vi "Step Forward.vi"(3 "error in":errorcluster, 4 "Data in":T1, 5 "Step control reference in":refnum<vi>) -> (0 "error out":errorcluster, 1 "Data out":T1, 2 "Step control reference out":refnum<vi>)   [LabVIEW 2015]
uses:
  Data.ctl
  Diagnostics.ctl
  Systems.ctl
  Step Vis/Steps.lvlib
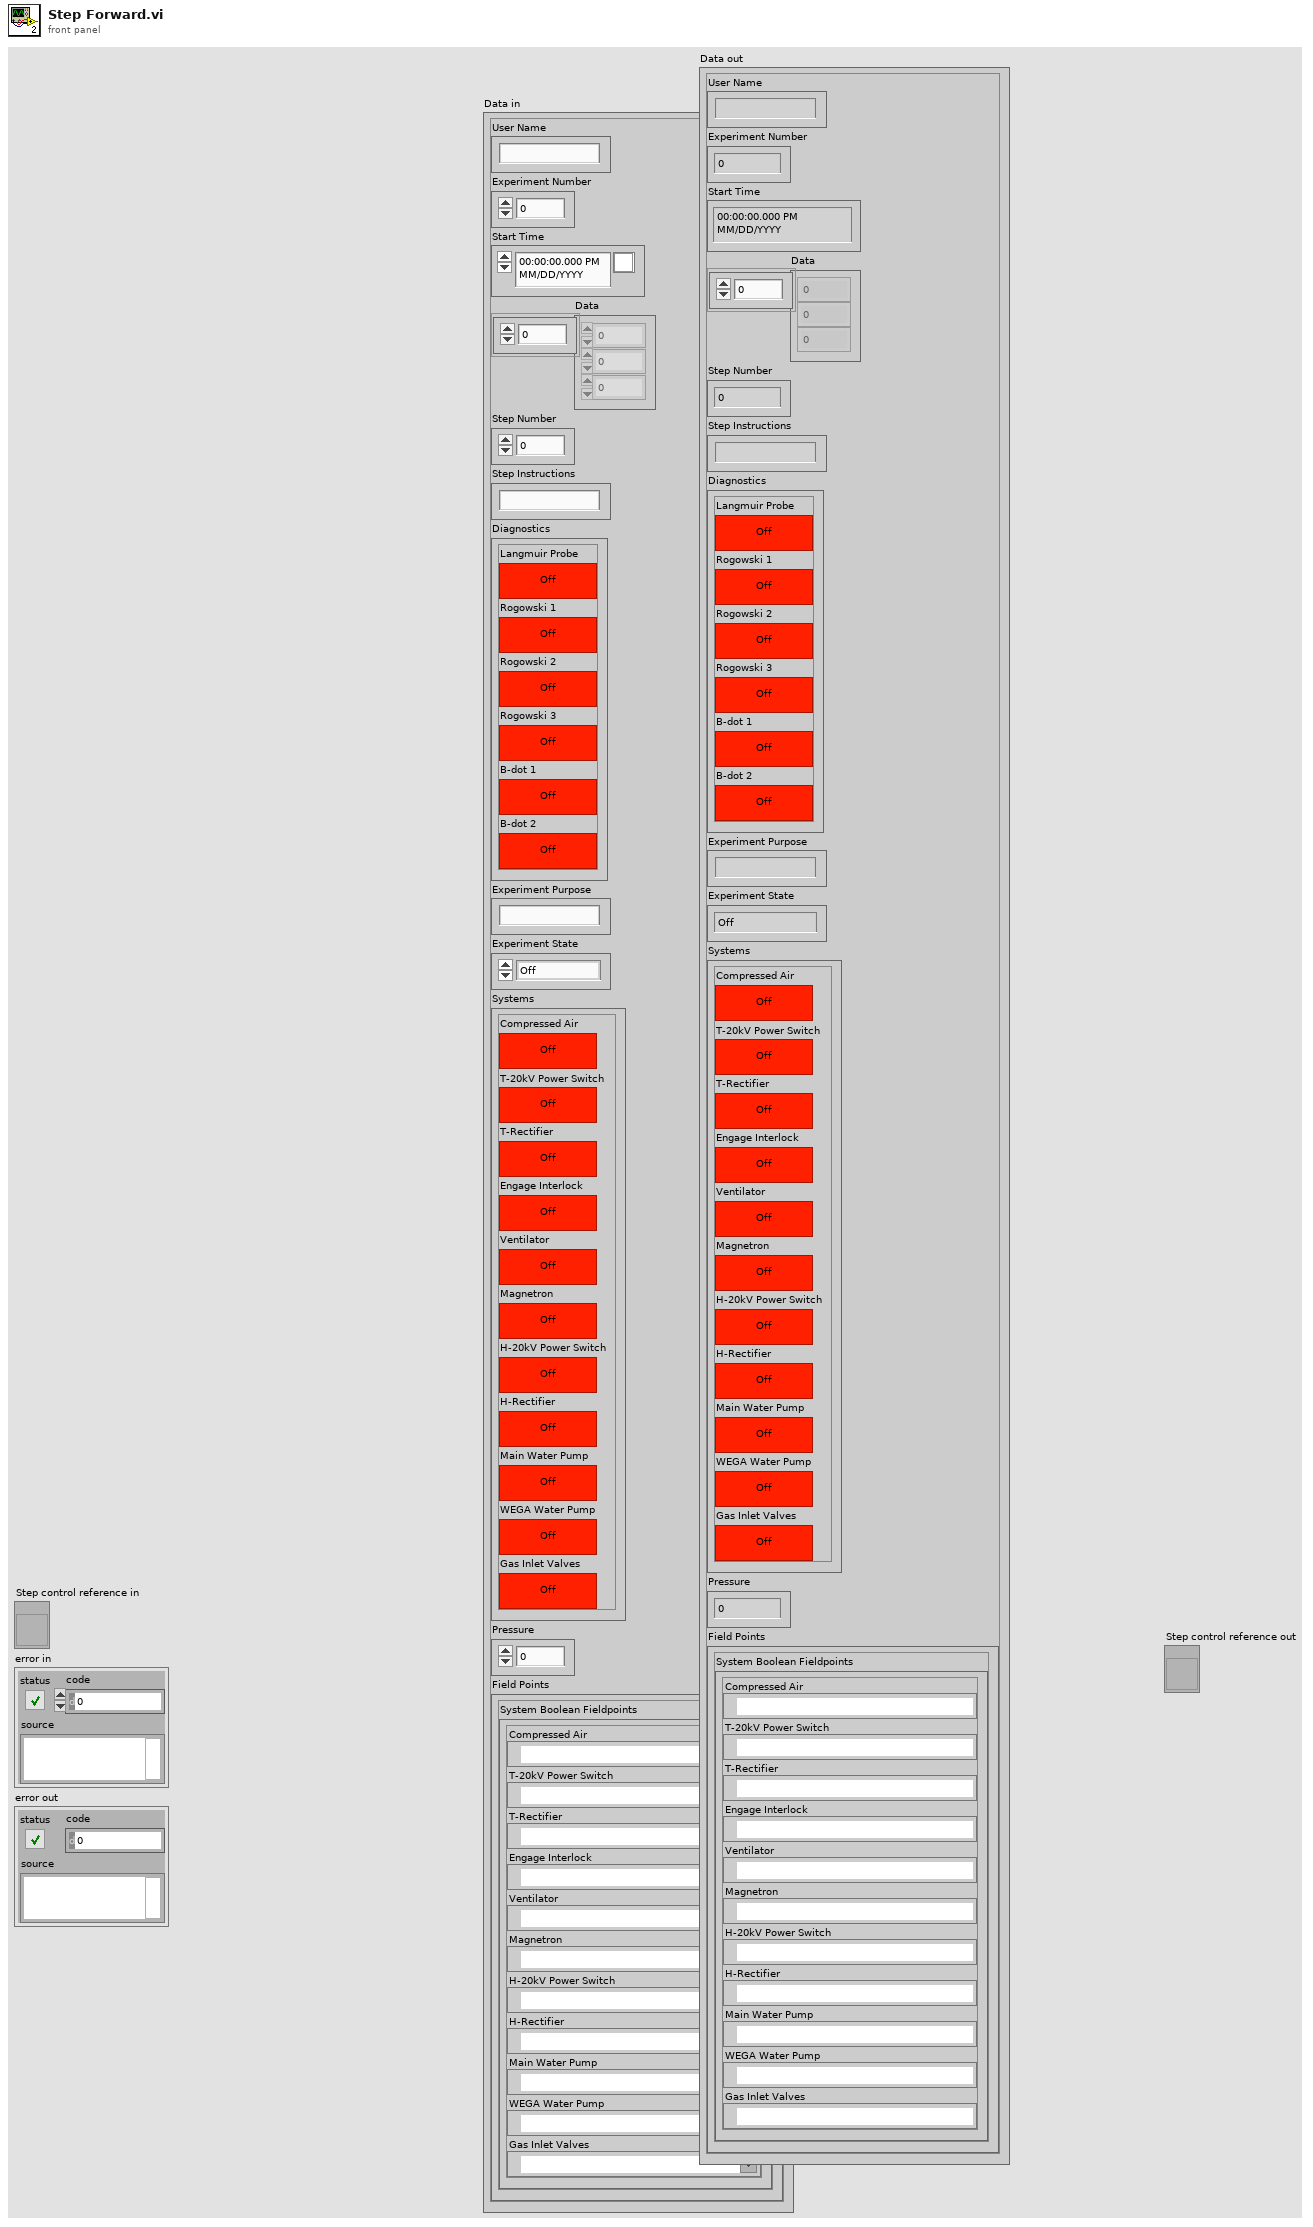
[diagram p1: front panel]
types:
  T1 = typedef "Data.ctl" = cluster{"User Name":string, "Experiment Number":i32, "Start Time":timestamp, "Data":dbl[], "Step Number":i32, "Step Instructions":string, "Diagnostics":T2, "Experiment Purpose":string, "Experiment State":enum16{"Off", "Setting Up", "Ready", "In Progress", "Shutting Down"}, "Systems":T3, "Pressure":dbl, "Field Points":cluster{"System Boolean Fieldpoints":cluster{"Compressed Air":refnum<k21>, "T-20kV Power Switch":refnum<k21>, "T-Rectifier":refnum<k21>, "Engage Interlock":refnum<k21>, "Ventilator":refnum<k21>, "Magnetron":refnum<k21>, "H-20kV Power Switch":refnum<k21>, "H-Rectifier":refnum<k21>, "Main Water Pump":refnum<k21>, "WEGA Water Pump":refnum<k21>, "Gas Inlet Valves":refnum<k21>}}}
  T2 = typedef "Diagnostics.ctl" = cluster{"Langmuir Probe":bool, "Rogowski 1":bool, "Rogowski 2":bool, "Rogowski 3":bool, "B-dot 1":bool, "B-dot 2":bool}
  T3 = typedef "Systems.ctl" = cluster{"Compressed Air":bool, "T-20kV Power Switch":bool, "T-Rectifier":bool, "Engage Interlock":bool, "Ventilator":bool, "Magnetron":bool, "H-20kV Power Switch":bool, "H-Rectifier":bool, "Main Water Pump":bool, "WEGA Water Pump":bool, "Gas Inlet Valves":bool}
  T4 = enum16{"Off", "Setting Up", "Ready", "In Progress", "Shutting Down"}
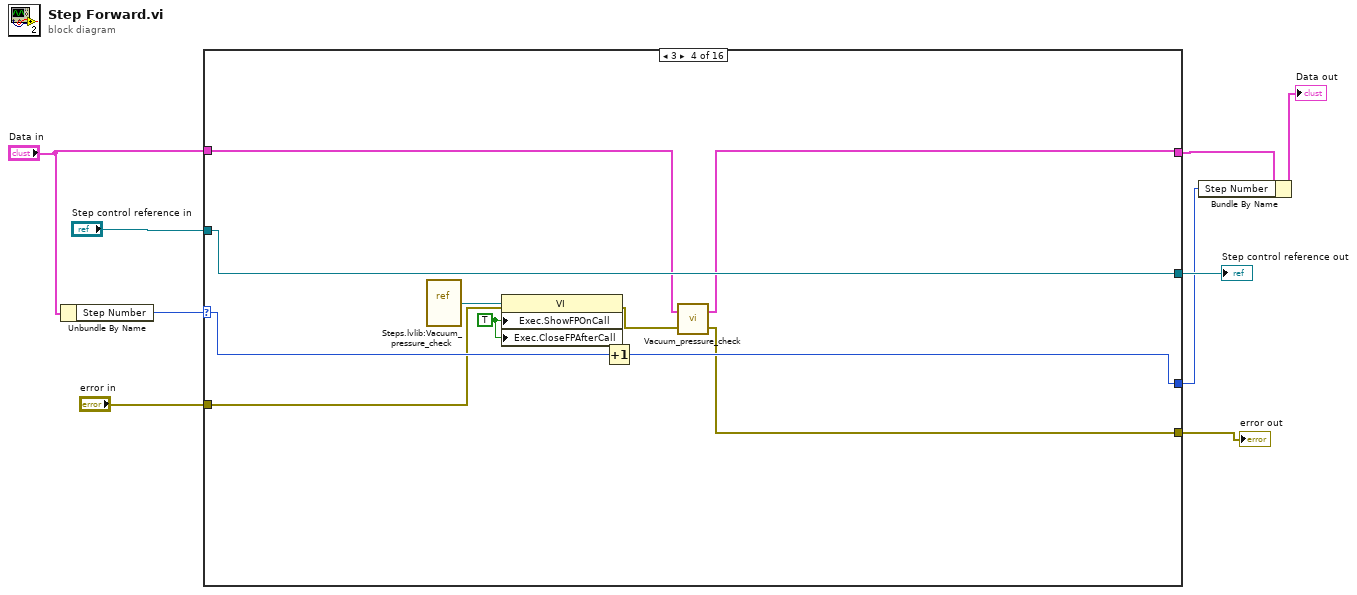
[diagram p0: block diagram]
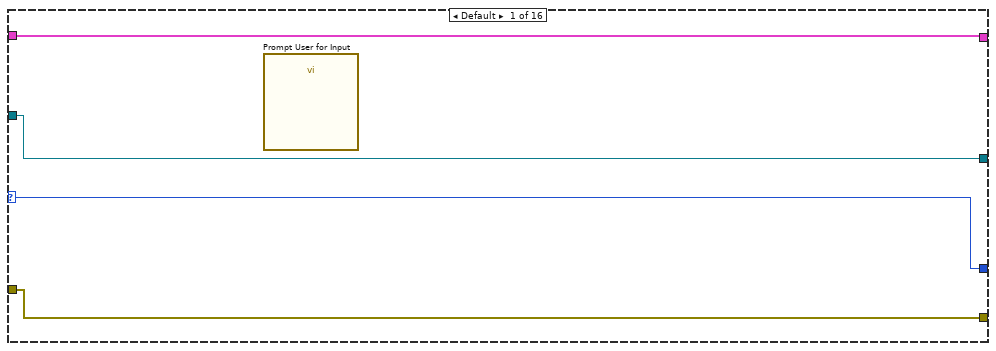
[diagram p2: hidden frame]
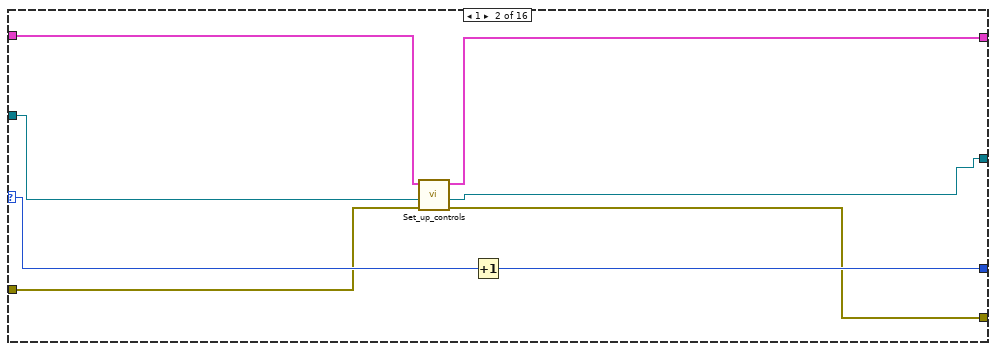
[diagram p3: hidden frame]
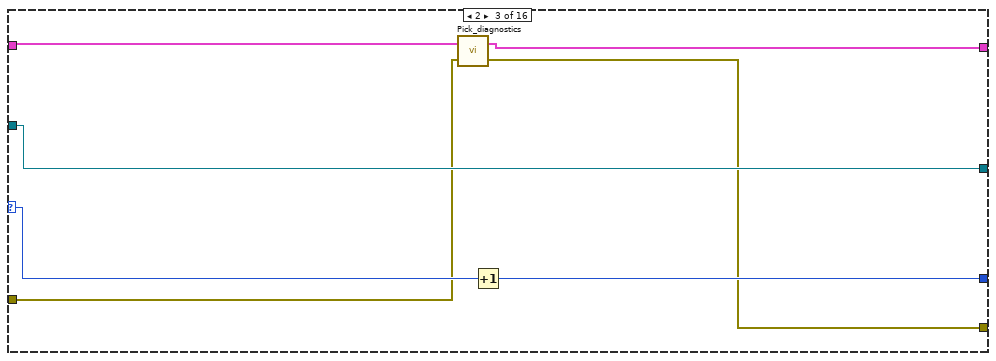
[diagram p4: hidden frame]
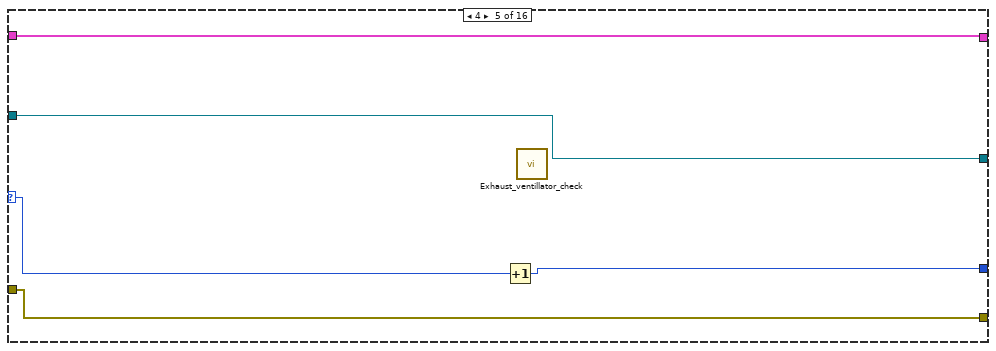
[diagram p5: hidden frame]
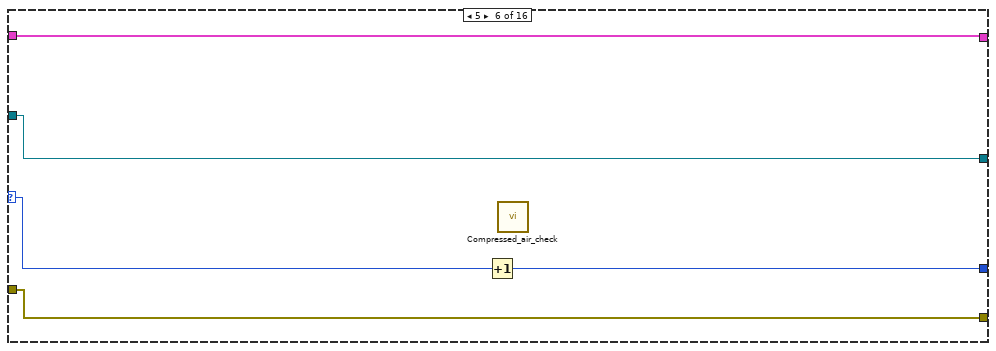
[diagram p6: hidden frame]
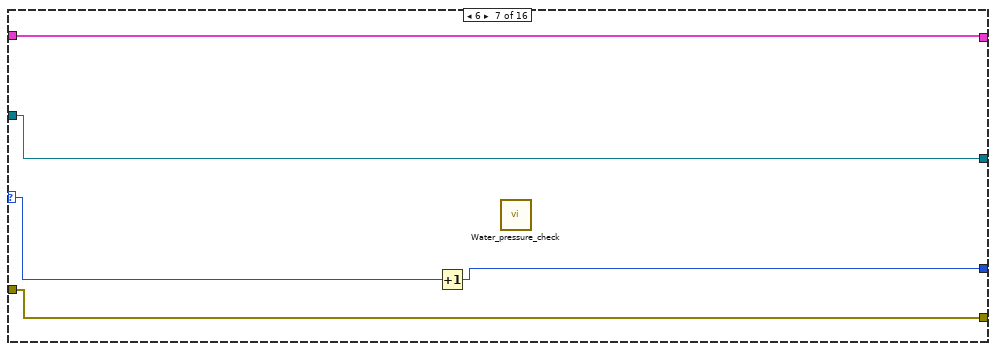
[diagram p7: hidden frame]
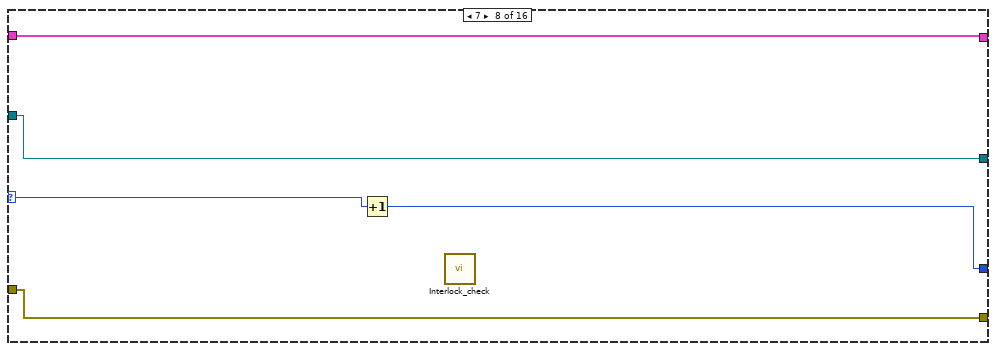
[diagram p8: hidden frame]
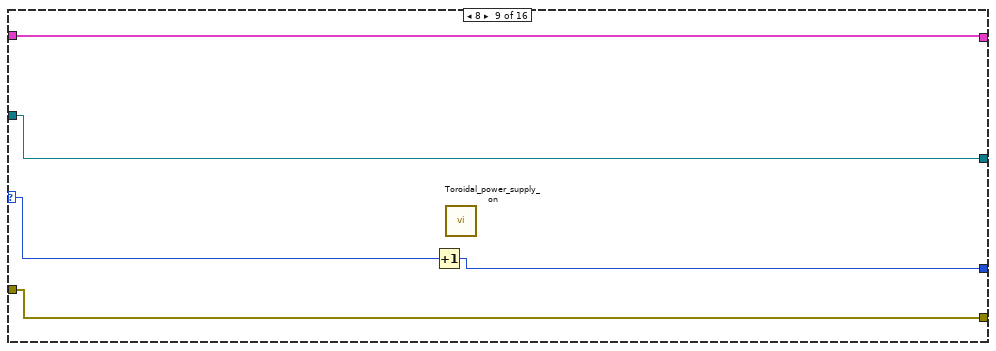
[diagram p9: hidden frame]
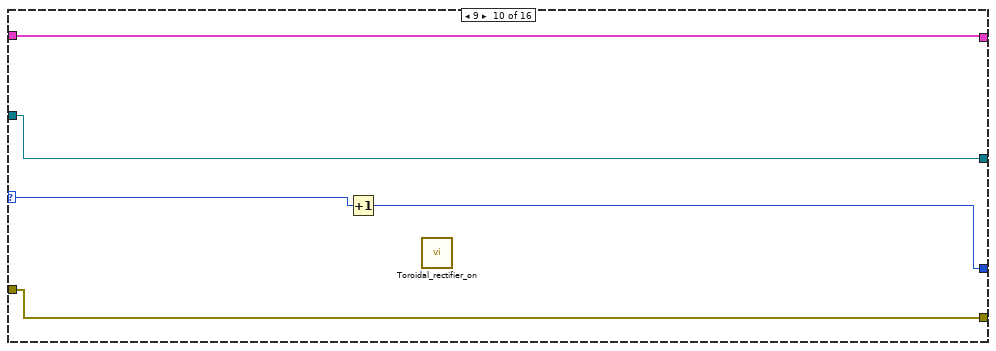
[diagram p10: hidden frame]
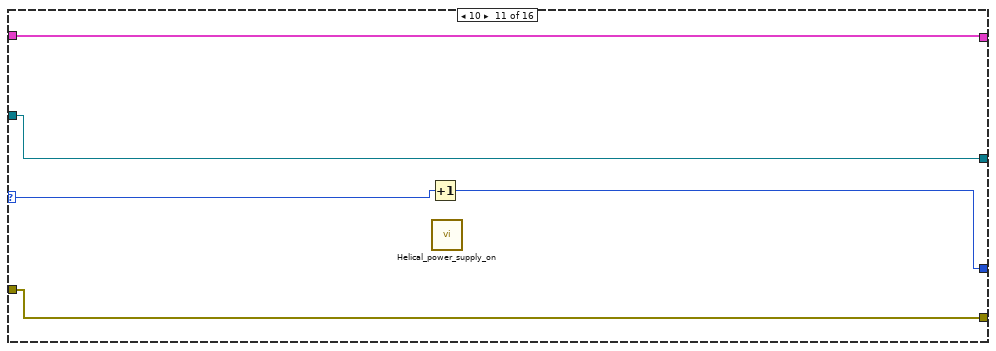
[diagram p11: hidden frame]
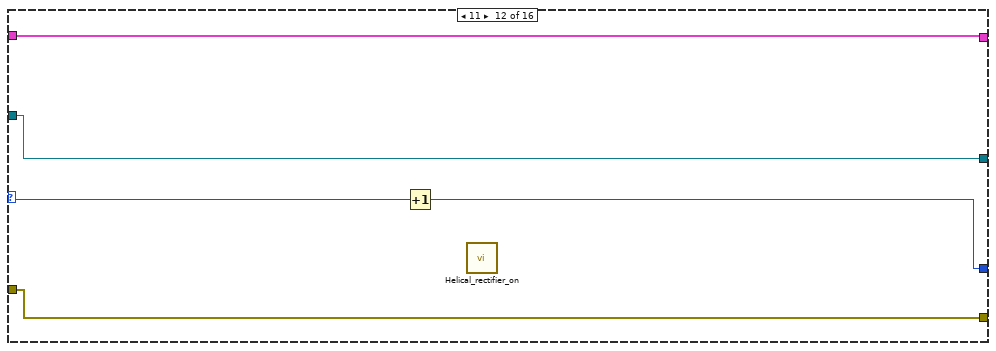
[diagram p12: hidden frame]
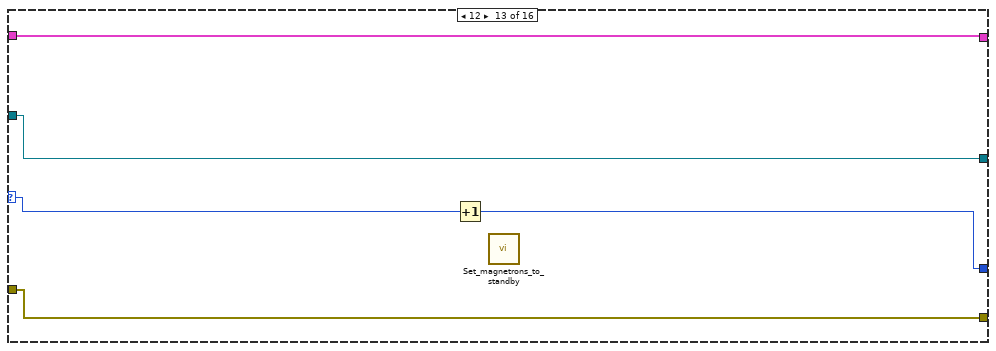
[diagram p13: hidden frame]
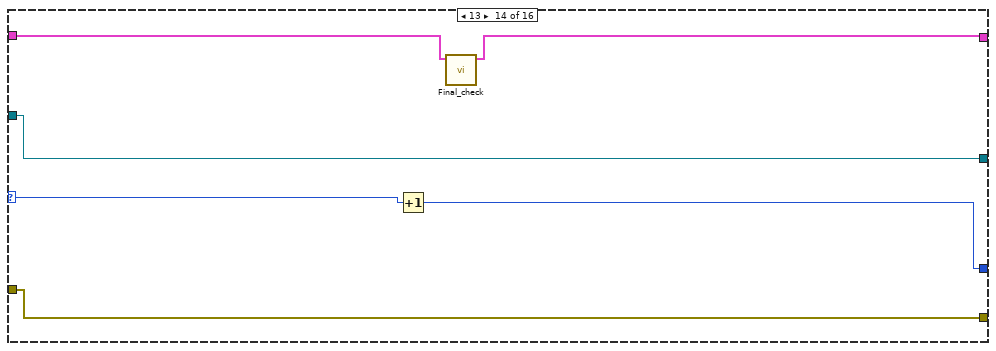
[diagram p14: hidden frame]
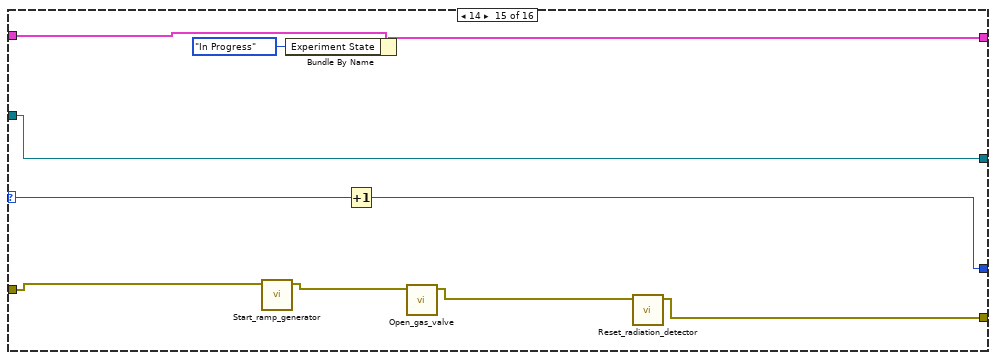
[diagram p15: hidden frame]
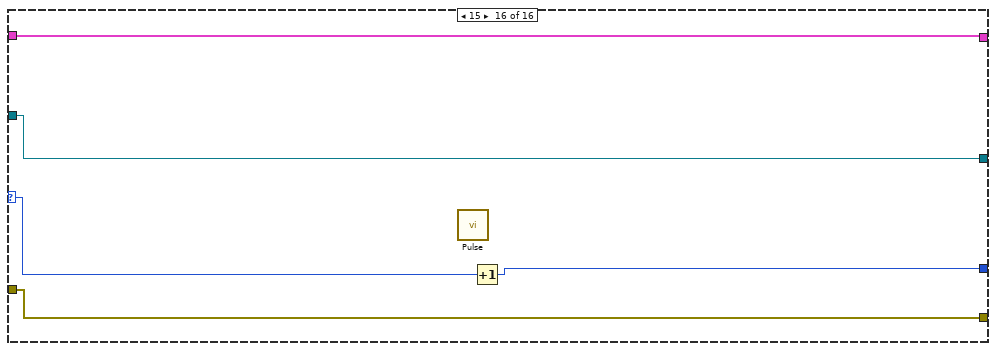
[diagram p16: hidden frame]
diagram:
  n1 = Unbundle By Name("Data in") -> ("Step Number"=w5:i32)
  n2 = case shown="3" w5 {
    selector: w5 -> [w12 w21 w28 w37 w39 w44 w49 w55 w59 w65 w70 w75 w79 w87 w97 w100]
    tunnel: "Step control reference in" -> [w13 w17 w26 w38 w41 w48 w53 w58 w63 w68 w73 w78 w83 w89 w99 w104]
    tunnel: [w13 w14 w26 w38 w41 w48 w53 w58 w63 w68 w73 w78 w83 w89 w99 w104] -> w8
    tunnel: [w12 w20 w27 w36 w40 w45 w50 w54 w60 w64 w69 w74 w80 w86 w98 w101] -> w3
    tunnel: "error in" -> [w11 w19 w25 w34 w43 w47 w52 w57 w62 w67 w72 w77 w82 w88 w96 w103]
    tunnel: [w11 w18 w24 w30 w43 w47 w52 w57 w62 w67 w72 w77 w82 w88 w93 w103] -> w6
    tunnel: "Data in" -> [w10 w16 w23 w32 w42 w46 w51 w56 w61 w66 w71 w76 w81 w85 w92 w102]
    tunnel: [w10 w15 w22 w31 w42 w46 w51 w56 w61 w66 w71 w76 w81 w84 w91 w102] -> w4
    frame Default {
      n3 = call "Prompt User for Input"() -> ()  [unwired: 18 in, 2 out]
    }
    frame 1 {
      n4 = call "Set_up_controls.vi"("error in"=w19, "reference"=w17, "Data in"=w16) -> ("error out"=w18:errorcluster, "reference out"=w14:refnum<vi>, "Data out"=w15:T1)  [unwired: 1 in, 1 out]
      n5 = Increment(x=w21) -> (x+1=w20:i32)
    }
    frame 2 {
      n6 = call "Pick_diagnostics.vi"("error in (no error)"=w25, "Data In"=w23) -> ("error out"=w24:errorcluster, "Data Out"=w22:T1)
      n7 = Increment(x=w28) -> (x+1=w27:i32)
    }
    frame 3 {
      w29 = TRUE ("Execution:Show Front Panel On Call")
      n8 = vi-ref "Steps.lvlib:Vacuum_pressure_check.vi"() -> (w35:refnum<vi>)
      n9 = property class="VI"(reference=w35, error in=w34, "Exec.ShowFPOnCall"=w29, "Exec.CloseFPAfterCall"=w29) -> (error out=w33:errorcluster)  [unwired: 1 out]
      n10 = Increment(x=w37) -> (x+1=w36:i32)
      n11 = call "Vacuum_pressure_check.vi"("error in"=w33, "Data in"=w32) -> ("error out"=w30:errorcluster, "Data out"=w31:T1)
    }
    frame 4 {
      n12 = Increment(x=w39) -> (x+1=w40:i32)
      n13 = call "Exhaust_ventillator_check.vi"() -> ()  [unwired: 12 in]
    }
    frame 5 {
      n14 = Increment(x=w44) -> (x+1=w45:i32)
      n15 = call "Compressed_air_check.vi"() -> ()  [unwired: 12 in]
    }
    frame 6 {
      n16 = Increment(x=w49) -> (x+1=w50:i32)
      n17 = call "Water_pressure_check.vi"() -> ()  [unwired: 12 in]
    }
    frame 7 {
      n18 = Increment(x=w55) -> (x+1=w54:i32)
      n19 = call "Interlock_check.vi"() -> ()  [unwired: 12 in]
    }
    frame 8 {
      n20 = Increment(x=w59) -> (x+1=w60:i32)
      n21 = call "Toroidal_power_supply_on.vi"() -> ()  [unwired: 12 in]
    }
    frame 9 {
      n22 = Increment(x=w65) -> (x+1=w64:i32)
      n23 = call "Toroidal_rectifier_on.vi"() -> ()  [unwired: 12 in]
    }
    frame 10 {
      n24 = Increment(x=w70) -> (x+1=w69:i32)
      n25 = call "Helical_power_supply_on.vi"() -> ()  [unwired: 12 in]
    }
    frame 11 {
      n26 = Increment(x=w75) -> (x+1=w74:i32)
      n27 = call "Helical_rectifier_on.vi"() -> ()  [unwired: 12 in]
    }
    frame 12 {
      n28 = Increment(x=w79) -> (x+1=w80:i32)
      n29 = call "Set_magnetrons_to_standby.vi"() -> ()  [unwired: 12 in]
    }
    frame 13 {
      n30 = Increment(x=w87) -> (x+1=w86:i32)
      n31 = call "Final_check.vi"("Data in"=w85) -> ("Data out"=w84:T1)  [unwired: 10 in]
    }
    frame 14 {
      n32 = call "Start_ramp_generator.vi"("error in"=w96) -> ("error out"=w95:errorcluster)  [unwired: 10 in]
      n33 = Bundle By Name(cluster=w92, "Experiment State"=T4."In Progress") -> (w91:T1)
      n34 = Increment(x=w97) -> (x+1=w98:i32)
      n35 = call "Open_gas_valve.vi"("error in"=w95) -> ("error out"=w94:errorcluster)  [unwired: 10 in]
      n36 = call "Reset_radiation_detector.vi"("error in"=w94) -> ("error out"=w93:errorcluster)  [unwired: 10 in]
    }
    frame 15 {
      n37 = call "Pulse.vi"() -> ()  [unwired: 12 in]
      n38 = Increment(x=w100) -> (x+1=w101:i32)
    }
  }
  "Step control reference out" <- w8
  "error out" <- w6
  n39 = Bundle By Name(cluster=w4, "Step Number"=w3) -> (→"Data out":T1)
